vi "Write_Instr.vi"(8 "error in (no error)":errorcluster caption="entrée d'erreur (pas d'erreur)", 11 "Class Relay_Board en entrée":refnum<class "Class Instrument UART.lvclass">) -> (0 "error out":errorcluster caption="sortie d'erreur", 3 "Class Relay_Board en Sortie":refnum<class "Class Instrument UART.lvclass">)   [LabVIEW 2020, in "Library Instrument & Equipement.lvlib" / "Library Instruments.lvlib" / "Class Instrument UART.lvclass"]
uses:
  Class Instrument UART.lvclass
  Class Instrument UART.lvclass/Class Instrument UART.ctl
  Instrument (Default)/Class Instrument (Default).lvclass
  UART/UART (Default)/Class UART (Default).lvclass
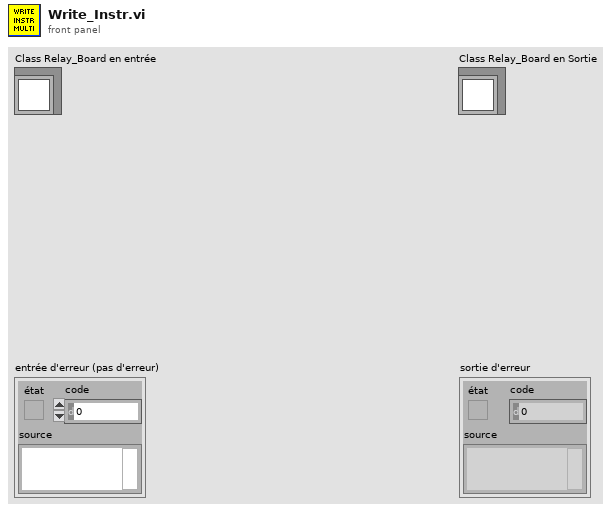
[diagram p1: front panel]
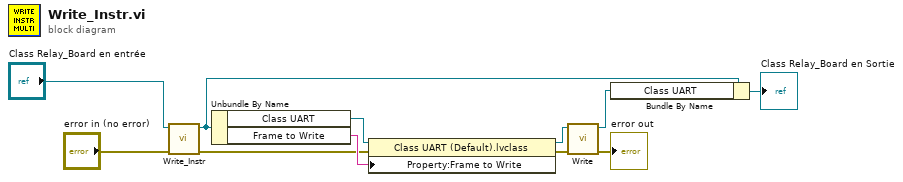
[diagram p0: block diagram]
diagram:
  n1 = call-parent "Write_Instr.vi"("error in (no error)"="error in (no error)", "Class Multimeter (Default) en entrée"="Class Relay_Board en entrée") -> ("error out"=w3:errorcluster, "Class Multimeter (Default) en sortie"=w9:refnum<class "Class Instrument UART.lvclass">)  [unwired: 8 in]
  n2 = Unbundle By Name(w9) -> ("Class UART"=w6:refnum<class "Class UART (Default).lvclass">, "Frame to Write"=w4:string)
  n3 = property class="Class UART (Default).lvclass"(reference=w6, error in=w3, "Property:Frame to Write"=w4) -> (reference out=w1:refnum<class "Class UART (Default).lvclass">, error out=w2:errorcluster)
  n4 = call-dynamic "Write.vi"("error in (no error)"=w2, "Class UART (Default) en entrée"=w1) -> ("error out"=→"error out":errorcluster, "Class UART (Default) en sortie"=w5:refnum<class "Class UART (Default).lvclass">)  [unwired: 8 in]
  n5 = Bundle By Name(cluster=w9, "Class UART"=w5) -> (→"Class Relay_Board en Sortie":refnum<class "Class Instrument UART.lvclass">)
